vi "Minimum Jerk Trajectory.vi"(8 "total time":dbl, 11 "t (sec)":dbl) -> (1 "In Range?":bool, 3 "ref_x (mm)":dbl)   [LabVIEW 2021]
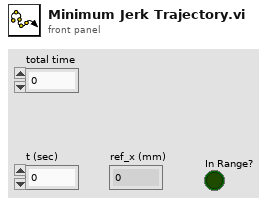
[diagram p1: front panel]
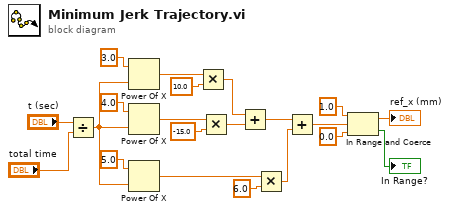
[diagram p0: block diagram]
diagram:
  n1 = Divide(x="t (sec)", y="total time") -> (x/y=w6:dbl)
  n2 = Power Of X(1:w6, 2:3.0 ("y")) -> (0:w10:dbl)
  n3 = Power Of X(1:w6, 2:4.0 ("y")) -> (0:w18:dbl)
  n4 = Power Of X(1:w6, 2:5.0 ("y")) -> (0:w17:dbl)
  n5 = Multiply(x=w10, y=10.0) -> (x*y=w14:dbl)
  n6 = Multiply(x=w18, y=-15.0) -> (x*y=w19:dbl)
  n7 = Add(x=w14, y=w19) -> (x+y=w21:dbl)
  n8 = Multiply(x=w17, y=6.0) -> (x*y=w20:dbl)
  n9 = Add(x=w21, y=w20) -> (x+y=w2:dbl)
  n10 = In Range and Coerce(upper limit=1.0, x=w2, lower limit=0.0) -> (coerced(x)=→"ref_x (mm)":dbl, In Range?=→"In Range?":bool)
